vi "PUBLIC.constructor.vi"(0 "name":string, 2 "data in":string, 5 "error in(no error)":errorcluster) -> (14 "i ref out":refnum<vi>, 16 "data out":string, 19 "error out":errorcluster)   [LabVIEW 2014]
doc: "This is the constructor of a class.\n\nLicense Agreement for this software:\n\nCopyright (C)\nGesellschaft für Schwerionenforschung, GSI\nPlanckstr. 1\n64291 Darmstadt\nGermany\n\nContact: D.Beck@gsi.de \n\nThis program is free software; you can redistribute it and/or modify it under the terms of the \nGNU General Public License as published by the Free Software Foundation; either version 2 of \nthe license, or (at your option) any later version.\n\nThis program is distributed in the hope that it will be useful, but WITHOUT ANY WARRANTY; \nwithout even the implied warranty of MERCHANTABILITY or FITNESS FOR A PARTICULAR PURPOSE. See the GNU General License for more details (http://www.gnu.org).\n\nGesellschaft für Schwerionenforschung, GSI\nPlanckstr. 1, 64291 Darmstadt, Germany\nFor all questions and ideas contact: M.Richter@gsi.de, H.Brand@gsi.de or D.Beck@gsi.de.\nLast update: 16-JUN-2004"
uses:
  CSCore/CSSystem/CSSystemLib/CSSystemLib.lvlib
  CSCore/CSApplicationBaseClasses/DeviceBase/DeviceBase.lvlib
  CSCore/CSApplicationBaseClasses/DeviceBase/DeviceBase.myEventNames.ctl
  Simple_DAQ_AnalogIO.lvlib
  CSCore/CSApplicationBaseClasses/PSChannelBase/PSChannelBase.lvlib
  CSCore/CSApplicationBaseClasses/PSChannelBase/PSChannelBase.myEventNames.ctl
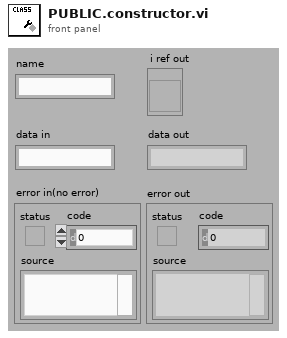
[diagram p1: front panel]
types:
  T1 = enum16{"SetAttribute", "GetAttribute", "CreateAttribute", "DestroyAttribute", "DestroyAllAtributes"}
  T2 = typedef "PSChannelBase.lvlib/PSChannelBase.myEventNames.ctl" = enum16{"lvmsg://EmergencyOff", "lvmsg://SetOnOff", "lvmsg://GetOnOff", "lvmsg://SetVoltage", "lvmsg://GetVoltage", "lvmsg://SetCurrent", "lvmsg://GetCurrent", "lvmsg://SetTripCurrent", "lvmsg://GetTripCurrent", "lvmsg://SetRampUpSpeed", "lvmsg://GetRampUpSpeed", "lvmsg://SetRampDownSpeed", "lvmsg://GetRampDownSpeed", "lvmsg://SetChannelOnOff", "lvmsg://GetChannelOnOff", "lvmsg://SetChannelVoltage", "lvmsg://GetChannelVoltage", "lvmsg://SetChannelCurrent", "lvmsg://GetChannelCurrent", "lvmsg://SetChannelTripCurrent", "lvmsg://GetChannelTripCurrent", "lvmsg://SetChannelRampUpSpeed", "lvmsg://GetChannelRampUpSpeed", "lvmsg://SetChannelRampDownSpeed", "lvmsg://GetChannelRampDownSpeed"}
  T3 = typedef "DeviceBase.lvlib/DeviceBase.myEventNames.ctl" = enum16{"lvmsg://Initialize", "lvmsg://Close", "lvmsg://Configure", "lvmsg://Reset", "lvmsg://IDQuery"}
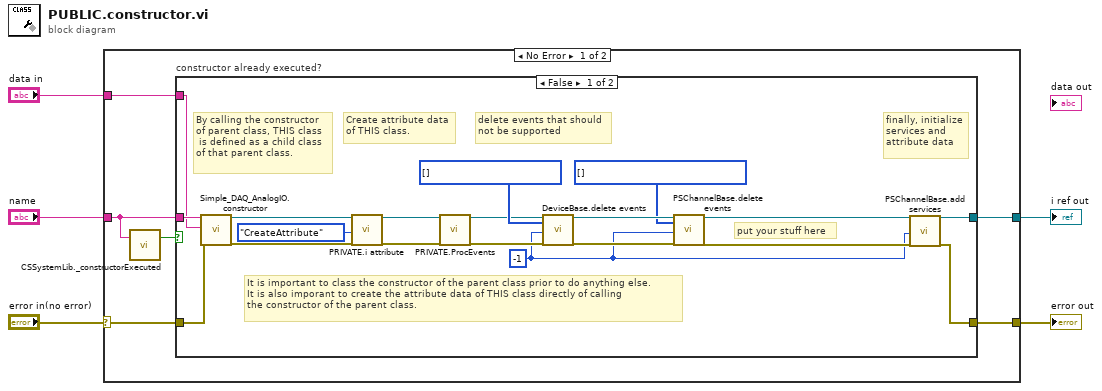
[diagram p0: block diagram]
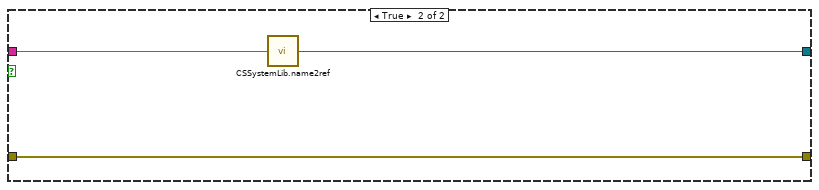
[diagram p2: hidden frame]
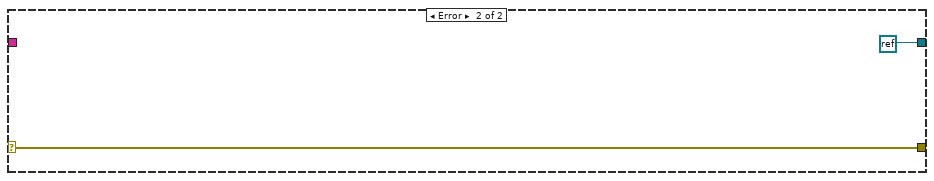
[diagram p3: hidden frame]
diagram:
  n1 = case shown="No Error" "error in(no error)" {
    selector: "error in(no error)" -> [w9 w34]
    tunnel: "name" -> [w8 _]
    tunnel: [w11 refnum<k0> refnum] -> w4
    tunnel: [w10 w34] -> w3
    tunnel: "data in" -> [w6 _]
    frame No Error {
      n2 = call "CSSystemLib._constructorExecuted.vi"("name"=w8) -> ("constructor executed?"=w7:bool)  [unwired: 18 in]
      n3 = case "constructor already executed?" shown="False" w7 {
        tunnel: w8 -> [w27 w33]
        tunnel: [w15 w32] -> w11
        tunnel: [w14 w31] -> w10
        tunnel: w9 -> [w24 w31]
        tunnel: w6 -> [w23 _]
        frame False {
          w17 = T2[] [] items=["lvmsg://EmergencyOff", "lvmsg://SetOnOff", "lvmsg://GetOnOff", "lvmsg://SetVoltage", "lvmsg://GetVoltage", "lvmsg://SetCurrent", "lvmsg://GetCurrent", "lvmsg://SetTripCurrent", "lvmsg://GetTripCurrent", "lvmsg://SetRampUpSpeed", "lvmsg://GetRampUpSpeed", "lvmsg://SetRampDownSpeed", "lvmsg://GetRampDownSpeed", "lvmsg://SetChannelOnOff", "lvmsg://GetChannelOnOff", "lvmsg://SetChannelVoltage", "lvmsg://GetChannelVoltage", "lvmsg://SetChannelCurrent", "lvmsg://GetChannelCurrent", "lvmsg://SetChannelTripCurrent", "lvmsg://GetChannelTripCurrent", "lvmsg://SetChannelRampUpSpeed", "lvmsg://GetChannelRampUpSpeed", "lvmsg://SetChannelRampDownSpeed", "lvmsg://GetChannelRampDownSpeed"] ("events")
          w22 = T3[] [] items=["lvmsg://Initialize", "lvmsg://Close", "lvmsg://Configure", "lvmsg://Reset", "lvmsg://IDQuery"] ("events")
          w12 = -1 ("ms timeout (10000)")
          # "finally, initialize\nservices and\nattribute data"
          # "put your stuff here"
          # "delete events that should\nnot be supported"
          # "It is important to class the constructor of the parent class prior to do anything else.\nIt is also imporant to create the attribute data of THIS class directly of calling\nthe constructor of the parent class."
          # "Create attribute data\nof THIS class."
          # "By calling the constructor\nof parent class, THIS class\n is defined as a child class\nof that parent class."
          n4 = call "Simple_DAQ_AnalogIO.constructor.vi"("name"=w27, "data in"=w23, "error in(no error)"=w24) -> ("i ref out"=w30:refnum<vi>, "error out"=w29:errorcluster)  [unwired: 14 in, 1 out]
          n5 = call "PRIVATE.i attribute.vi"("VI Refnum"=w30, "Action"=T1."CreateAttribute", "error in (no error)"=w29) -> ("VI Refnum out"=w26:refnum<vi>, "error out"=w25:errorcluster)  [unwired: 14 in, 1 out]
          n6 = call "PRIVATE.ProcEvents.vi"("i ref in"=w26, "error in"=w25) -> ("i ref out"=w21:refnum<vi>, "error out"=w20:errorcluster)  [unwired: 16 in]
          n7 = call "DeviceBase.delete events.vi"("i ref in"=w21, "events"=w22, "ms timeout (10000)"=w12, "error in (no error)"=w20) -> ("i ref out"=w19:refnum<vi>, "error out"=w18:errorcluster)  [unwired: 13 in, 1 out]
          n8 = call "PSChannelBase.delete events.vi"("i ref in"=w19, "events"=w17, "ms timeout (10000)"=w12, "error in (no error)"=w18) -> ("i ref out"=w16:refnum<vi>, "error out"=w13:errorcluster)  [unwired: 13 in, 1 out]
          n9 = call "PSChannelBase.add services.vi"("i ref in"=w16, "ms timeout (10000)"=w12, "error in (no error)"=w13) -> ("i ref out"=w15:refnum<vi>, "error out"=w14:errorcluster)  [unwired: 14 in, 1 out]
        }
        frame True {
          n10 = call "CSSystemLib.name2ref.vi"("name"=w33) -> ("obj refnum"=w32:refnum<vi>)
        }
      }
    }
    frame Error {
    }
  }
  "i ref out" <- w4
  "error out" <- w3
